vi "_old_update_material_and_process.vi"   [LabVIEW 2018]
uses:
  float_format_codes.ctl
types:
  T1 = typedef "float_format_codes.ctl" = enum16{"REAL_3F20 X.XX", "REAL_3F20 XX.X", "REAL_3F20 XXX", "REAL_3X1", "REAL_4F21 XX.XX", "REAL_4F21 XXX.X", "REAL_4F31 X.XXX", "REAL_4F31 XX.XX", "REAL_4F31 XXX.X", "REAL_4X1", "REAL_4X2", "REAL_4X3", "REAL_5F32 XX.XXX", "REAL_5F32 XXX.XX", "REAL_5X2", "REAL_5X3", "REAL_6F32 XXX.XXX", "REAL_6F32 XXXX.XX"}
  T2 = cluster{"Process number":u8, "Layer number":u8, "Parameter":u8}
  T3 = cluster{"Process number":u8, "Layer number":u8, "Parameter":dbl}
  T4 = cluster{"Process number":u8, "Layer number":u8, "Parameter":bool}
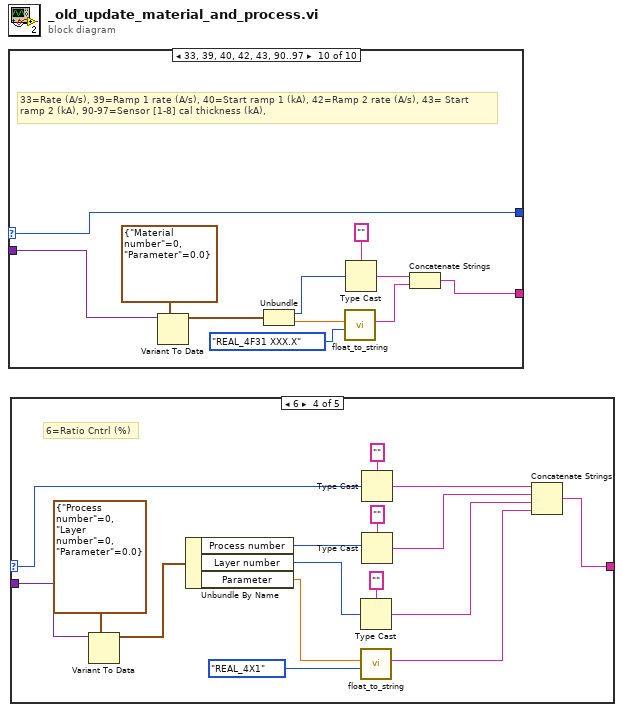
[diagram p0: block diagram]
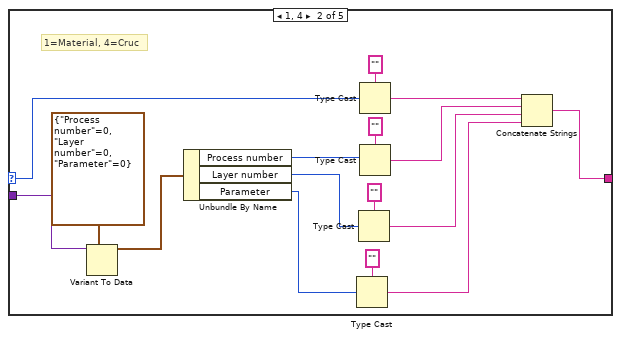
[diagram p3: hidden frame]
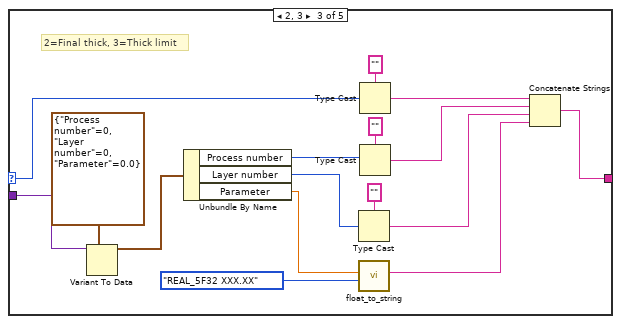
[diagram p4: hidden frame]
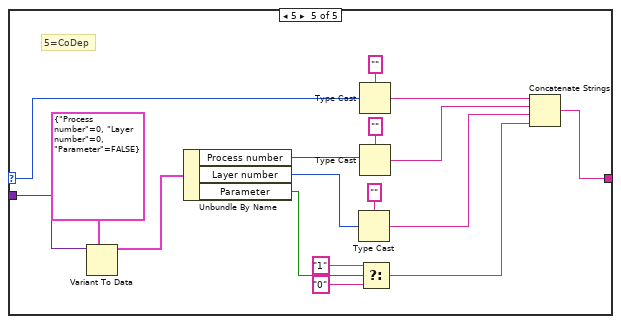
[diagram p5: hidden frame]
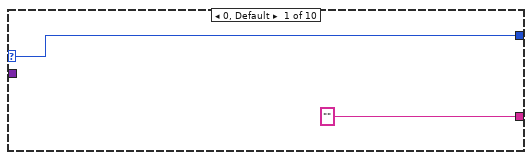
[diagram p6: hidden frame]
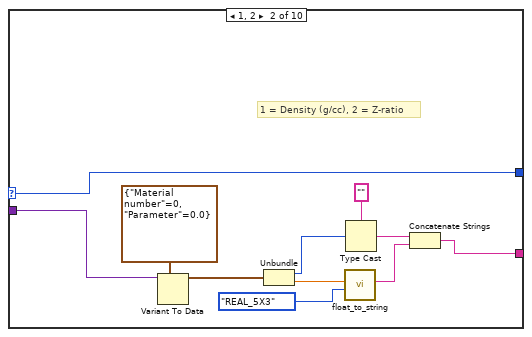
[diagram p7: hidden frame]
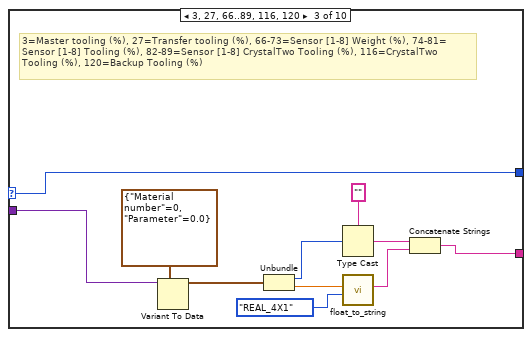
[diagram p8: hidden frame]
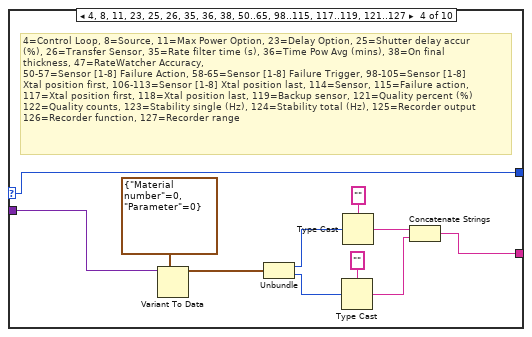
[diagram p9: hidden frame]
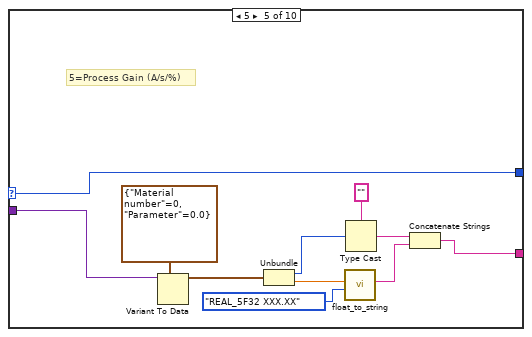
[diagram p10: hidden frame]
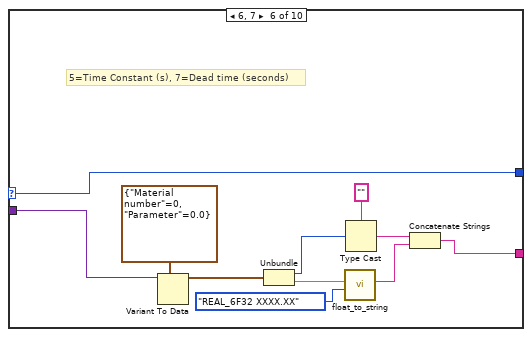
[diagram p11: hidden frame]
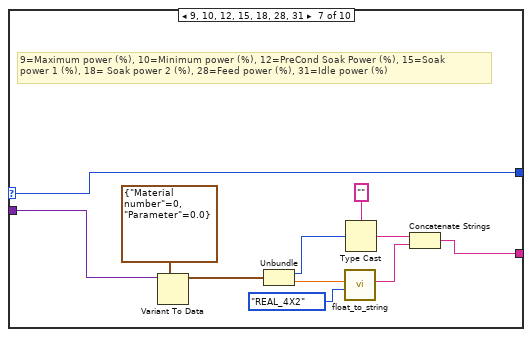
[diagram p12: hidden frame]
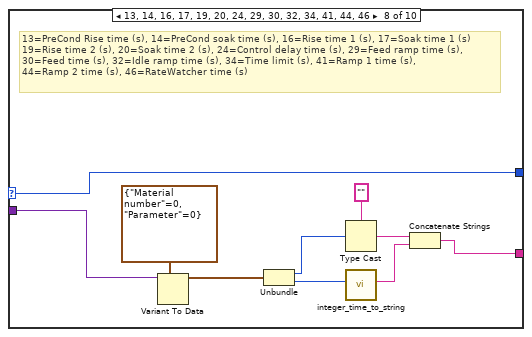
[diagram p13: hidden frame]
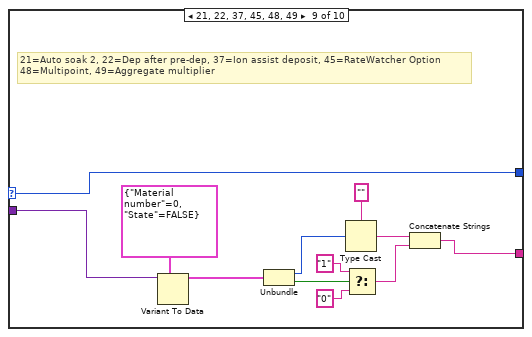
[diagram p14: hidden frame]
diagram:
  n1 = case shown="33, 39, 40, 42, 43, 90..97" {
    selector: _ -> [w1 w6 w17 w25 w39 w50 w61 w71 w83 w94]
    tunnel: ["" w7 w18 w29 w40 w51 w62 w72 w84 w95] -> _
    tunnel: _ -> [_ w8 w19 w30 w41 w52 w63 w73 w85 w96]
    tunnel: [w1 w6 w17 w25 w39 w50 w61 w71 w83 w94] -> _
    frame 0, Default {
    }
    frame 1, 2 {
      # "1 = Density (g/cc), 2 = Z-ratio"
      n2 = Variant To Data(type=cluster{"Material number":u8, "Parameter":sgl} {"Material number"=0, "Parameter"=0.0}, Variant=w8) -> (data=w11:cluster{"Material number":u8, "Parameter":sgl})  [unwired: 1 in, 1 out]
      n3 = Unbundle(w11) -> ("Material number"=w12:u8, "Parameter"=w4:sgl)
      n4 = call "float_to_string.vi"("Float format"=float_format_codes."REAL_5X3", "Float"=w4) -> ("String"=w3:string)  [unwired: 9 in]
      n5 = Type Cast(type="", x=w12) -> (*(type *) &x=w13:string)
      n6 = Concatenate Strings(w13, w3) -> (w7:string)
    }
    frame 3, 27, 66..89, 116, 120 {
      # "3=Master tooling (%), 27=Transfer tooling (%), 66-73=Sensor [1-8] Weight (%), 74-81=\nSensor [1-8] Tooling (%), 82-89=Sensor [1-8] CrystalTwo Tooling (%), 116=CrystalTwo\nTooling (%), 120=Backup Tooling (%)"
      n7 = Variant To Data(type=cluster{"Material number":u8, "Parameter":sgl} {"Material number"=0, "Parameter"=0.0}, Variant=w19) -> (data=w22:cluster{"Material number":u8, "Parameter":sgl})  [unwired: 1 in, 1 out]
      n8 = Unbundle(w22) -> ("Material number"=w23:u8, "Parameter"=w15:sgl)
      n9 = Type Cast(type="", x=w23) -> (*(type *) &x=w24:string)
      n10 = call "float_to_string.vi"("Float format"=float_format_codes."REAL_4X1", "Float"=w15) -> ("String"=w14:string)  [unwired: 9 in]
      n11 = Concatenate Strings(w24, w14) -> (w18:string)
    }
    frame 4, 8, 11, 23, 25, 26, 35, 36, 38, 50..65, 98..115, 117..119, 121..127 {
      # "4=Control Loop, 8=Source, 11=Max Power Option, 23=Delay Option, 25=Shutter delay accur\n(%), 26=Transfer Sensor, 35=Rate filter time (s), 36=Time Pow Avg (mins), 38=On final\nthickness, 47=RateWatcher Accuracy,\n50-57=Sensor [1-8] Failure Action, 58-65=Sensor [1-8] Failure Trigger, 98-105=Sensor [1-8]\nXtal position first, 106-113=Sensor [1-8] Xtal position last, 114=Sensor, 115=Failure action,\n117=Xtal position first, 118=Xtal position last, 119=Backup sensor, 121=Quality percent (%)\n122=Quality counts, 123=Stability single (Hz), 124=Stability total (Hz), 125=Recorder output\n126=Recorder function, 127=Recorder range"
      n12 = Variant To Data(type=cluster{"Material number":u8, "Parameter":u8} {"Material number"=0, "Parameter"=0}, Variant=w30) -> (data=w33:cluster{"Material number":u8, "Parameter":u8})  [unwired: 1 in, 1 out]
      n13 = Unbundle(w33) -> ("Material number"=w34:u8, "Parameter"=w27:u8)
      n14 = Type Cast(type="", x=w27) -> (*(type *) &x=w26:string)
      n15 = Type Cast(type="", x=w34) -> (*(type *) &x=w35:string)
      n16 = Concatenate Strings(w35, w26) -> (w29:string)
    }
    frame 5 {
      # "5=Process Gain (A/s/%)"
      n17 = Variant To Data(type=cluster{"Material number":u8, "Parameter":sgl} {"Material number"=0, "Parameter"=0.0}, Variant=w41) -> (data=w44:cluster{"Material number":u8, "Parameter":sgl})  [unwired: 1 in, 1 out]
      n18 = Unbundle(w44) -> ("Material number"=w45:u8, "Parameter"=w37:sgl)
      n19 = call "float_to_string.vi"("Float format"=float_format_codes."REAL_5F32 XXX.XX", "Float"=w37) -> ("String"=w36:string)  [unwired: 9 in]
      n20 = Type Cast(type="", x=w45) -> (*(type *) &x=w46:string)
      n21 = Concatenate Strings(w46, w36) -> (w40:string)
    }
    frame 6, 7 {
      # "5=Time Constant (s), 7=Dead time (seconds)"
      n22 = Variant To Data(type=cluster{"Material number":u8, "Parameter":sgl} {"Material number"=0, "Parameter"=0.0}, Variant=w52) -> (data=w55:cluster{"Material number":u8, "Parameter":sgl})  [unwired: 1 in, 1 out]
      n23 = Unbundle(w55) -> ("Material number"=w56:u8, "Parameter"=w48:sgl)
      n24 = call "float_to_string.vi"("Float format"=float_format_codes."REAL_6F32 XXXX.XX", "Float"=w48) -> ("String"=w47:string)  [unwired: 9 in]
      n25 = Type Cast(type="", x=w56) -> (*(type *) &x=w57:string)
      n26 = Concatenate Strings(w57, w47) -> (w51:string)
    }
    frame 9, 10, 12, 15, 18, 28, 31 {
      # "9=Maximum power (%), 10=Minimum power (%), 12=PreCond Soak Power (%), 15=Soak\npower 1 (%), 18= Soak power 2 (%), 28=Feed power (%), 31=Idle power (%)"
      n27 = Variant To Data(type=cluster{"Material number":u8, "Parameter":sgl} {"Material number"=0, "Parameter"=0.0}, Variant=w63) -> (data=w66:cluster{"Material number":u8, "Parameter":sgl})  [unwired: 1 in, 1 out]
      n28 = Unbundle(w66) -> ("Material number"=w67:u8, "Parameter"=w59:sgl)
      n29 = call "float_to_string.vi"("Float format"=float_format_codes."REAL_4X2", "Float"=w59) -> ("String"=w58:string)  [unwired: 9 in]
      n30 = Type Cast(type="", x=w67) -> (*(type *) &x=w68:string)
      n31 = Concatenate Strings(w68, w58) -> (w62:string)
    }
    frame 13, 14, 16, 17, 19, 20, 24, 29, 30, 32, 34, 41, 44, 46 {
      # "13=PreCond Rise time (s), 14=PreCond soak time (s), 16=Rise time 1 (s), 17=Soak time 1 (s)\n19=Rise time 2 (s), 20=Soak time 2 (s), 24=Control delay time (s), 29=Feed ramp time (s),\n30=Feed time (s), 32=Idle ramp time (s), 34=Time limit (s), 41=Ramp 1 time (s),\n44=Ramp 2 time (s), 46=RateWatcher time (s)"
      n32 = Variant To Data(type=cluster{"Material number":u8, "Parameter":u16} {"Material number"=0, "Parameter"=0}, Variant=w73) -> (data=w76:cluster{"Material number":u8, "Parameter":u16})  [unwired: 1 in, 1 out]
      n33 = Unbundle(w76) -> ("Material number"=w77:u8, "Parameter"=w69:u16)
      n34 = Type Cast(type="", x=w77) -> (*(type *) &x=w78:string)
      n35 = call "integer_time_to_string.vi"("Time (s)"=w69) -> ("Time string (mm:ss)"=w70:string)  [unwired: 9 in, 1 out]
      n36 = Concatenate Strings(w78, w70) -> (w72:string)
    }
    frame 21, 22, 37, 45, 48, 49 {
      # "21=Auto soak 2, 22=Dep after pre-dep, 37=Ion assist deposit, 45=RateWatcher Option\n48=Multipoint, 49=Aggregate multiplier"
      n37 = Variant To Data(type=cluster{"Material number":u8, "State":bool} {"Material number"=0, "State"=FALSE}, Variant=w85) -> (data=w88:cluster{"Material number":u8, "State":bool})  [unwired: 1 in, 1 out]
      n38 = Unbundle(w88) -> ("Material number"=w89:u8, "State"=w82:bool)
      n39 = Type Cast(type="", x=w89) -> (*(type *) &x=w90:string)
      n40 = Select(t="1", s=w82, f="0") -> (s? t:f=w81:string)
      n41 = Concatenate Strings(w90, w81) -> (w84:string)
    }
    frame 33, 39, 40, 42, 43, 90..97 {
      # "33=Rate (A/s), 39=Ramp 1 rate (A/s), 40=Start ramp 1 (kA), 42=Ramp 2 rate (A/s), 43= Start\nramp 2 (kA), 90-97=Sensor [1-8] cal thickness (kA),"
      n42 = Variant To Data(type=cluster{"Material number":u8, "Parameter":dbl} {"Material number"=0, "Parameter"=0.0}, Variant=w96) -> (data=w99:cluster{"Material number":u8, "Parameter":dbl})  [unwired: 1 in, 1 out]
      n43 = Unbundle(w99) -> ("Material number"=w100:u8, "Parameter"=w92:dbl)
      n44 = call "float_to_string.vi"("Float format"=float_format_codes."REAL_4F31 XXX.X", "Float"=w92) -> ("String"=w91:string)  [unwired: 9 in]
      n45 = Type Cast(type="", x=w100) -> (*(type *) &x=w101:string)
      n46 = Concatenate Strings(w101, w91) -> (w95:string)
    }
  }
  n47 = case shown="6" {
    selector: _ -> [_ w108 w125 w141 w158]
    tunnel: _ -> [_ w116 w132 w148 w165]
    tunnel: [_ w103 w121 w137 w154] -> _
    frame 0, Default {
    }
    frame 1, 4 {
      # "1=Material, 4=Cruc"
      n48 = Variant To Data(type=T2 {"Process number"=0, "Layer number"=0, "Parameter"=0}, Variant=w116) -> (data=w107:T2)  [unwired: 1 in, 1 out]
      n49 = Unbundle By Name(w107) -> ("Process number"=w106:u8, "Layer number"=w105:u8, "Parameter"=w104:u8)
      n50 = Type Cast(type="", x=w104) -> (*(type *) &x=w102:string)
      n51 = Type Cast(type="", x=w105) -> (*(type *) &x=w110:string)
      n52 = Type Cast(type="", x=w108) -> (*(type *) &x=w113:string)
      n53 = Type Cast(type="", x=w106) -> (*(type *) &x=w112:string)
      n54 = Concatenate Strings(w113, w112, w110, w102) -> (w103:string)
    }
    frame 2, 3 {
      # "2=Final thick, 3=Thick limit"
      n55 = Variant To Data(type=T3 {"Process number"=0, "Layer number"=0, "Parameter"=0.0}, Variant=w132) -> (data=w124:T3)  [unwired: 1 in, 1 out]
      n56 = Unbundle By Name(w124) -> ("Process number"=w123:u8, "Layer number"=w122:u8, "Parameter"=w120:dbl)
      n57 = Type Cast(type="", x=w122) -> (*(type *) &x=w126:string)
      n58 = call "float_to_string.vi"("Float format"=float_format_codes."REAL_5F32 XXX.XX", "Float"=w120) -> ("String"=w118:string)  [unwired: 9 in]
      n59 = Type Cast(type="", x=w125) -> (*(type *) &x=w129:string)
      n60 = Type Cast(type="", x=w123) -> (*(type *) &x=w128:string)
      n61 = Concatenate Strings(w129, w128, w126, w118) -> (w121:string)
    }
    frame 6 {
      # "6=Ratio Cntrl (%)"
      n62 = Variant To Data(type=T3 {"Process number"=0, "Layer number"=0, "Parameter"=0.0}, Variant=w148) -> (data=w140:T3)  [unwired: 1 in, 1 out]
      n63 = Unbundle By Name(w140) -> ("Process number"=w139:u8, "Layer number"=w138:u8, "Parameter"=w136:dbl)
      n64 = Type Cast(type="", x=w138) -> (*(type *) &x=w142:string)
      n65 = call "float_to_string.vi"("Float format"=float_format_codes."REAL_4X1", "Float"=w136) -> ("String"=w134:string)  [unwired: 9 in]
      n66 = Type Cast(type="", x=w141) -> (*(type *) &x=w145:string)
      n67 = Type Cast(type="", x=w139) -> (*(type *) &x=w144:string)
      n68 = Concatenate Strings(w145, w144, w142, w134) -> (w137:string)
    }
    frame 5 {
      # "5=CoDep"
      n69 = Variant To Data(type=T4 {"Process number"=0, "Layer number"=0, "Parameter"=FALSE}, Variant=w165) -> (data=w157:T4)  [unwired: 1 in, 1 out]
      n70 = Unbundle By Name(w157) -> ("Process number"=w156:u8, "Layer number"=w155:u8, "Parameter"=w153:bool)
      n71 = Type Cast(type="", x=w155) -> (*(type *) &x=w159:string)
      n72 = Type Cast(type="", x=w158) -> (*(type *) &x=w162:string)
      n73 = Type Cast(type="", x=w156) -> (*(type *) &x=w161:string)
      n74 = Select(t="1", s=w153, f="0") -> (s? t:f=w150:string)
      n75 = Concatenate Strings(w162, w161, w159, w150) -> (w154:string)
    }
  }
